vi "save log.vi"(4 "camera":bool, 5 "auto/man":bool, 6 "projector":bool, 7 "disc":bool, 8 "Error in":errorcluster, 10 "Case Num":u32, 11 "Disc Number":string="Disc 26") -> (0 "Error out":errorcluster)   [LabVIEW 2019, in "database.lvlib"]
uses:
  database.lvlib
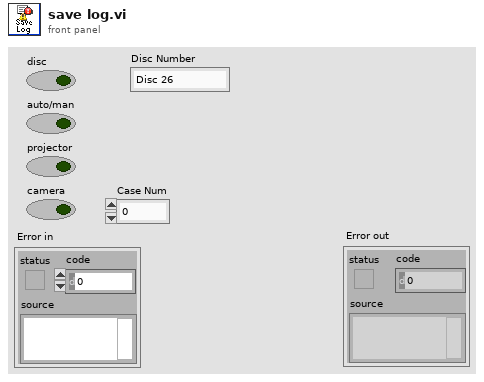
[diagram p1: front panel]
types:
  T1 = cluster{"f":string, "date/time string":string, "date/time string":string, "Disc Number":string}
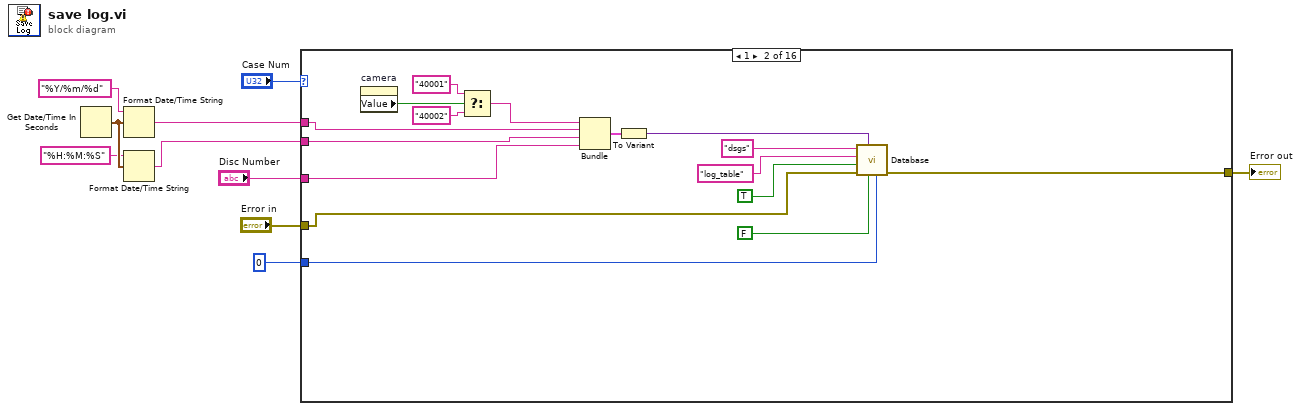
[diagram p0: block diagram]
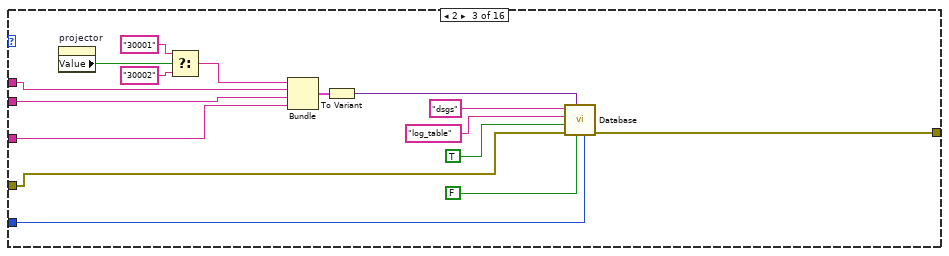
[diagram p3: hidden frame]
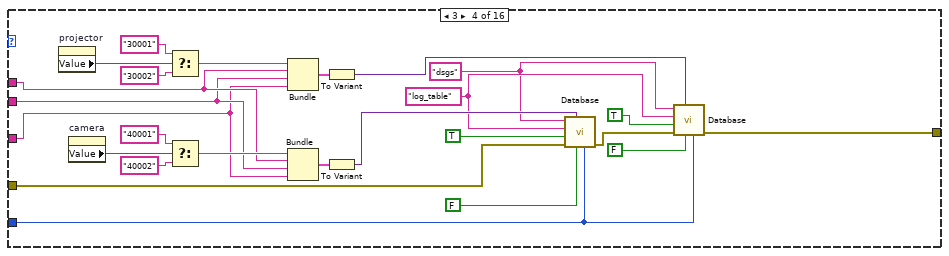
[diagram p4: hidden frame]
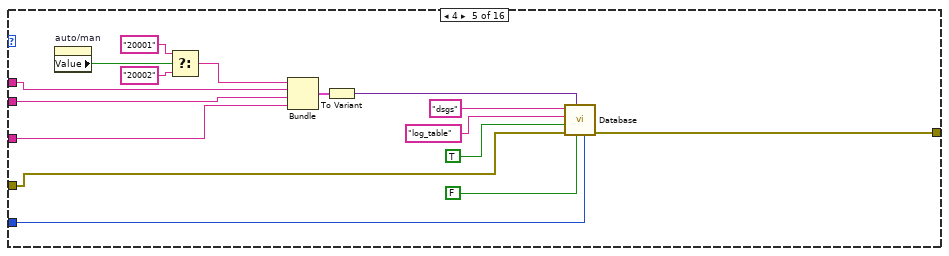
[diagram p5: hidden frame]
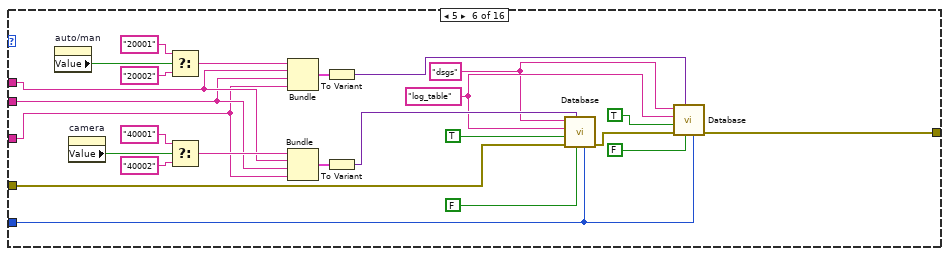
[diagram p6: hidden frame]
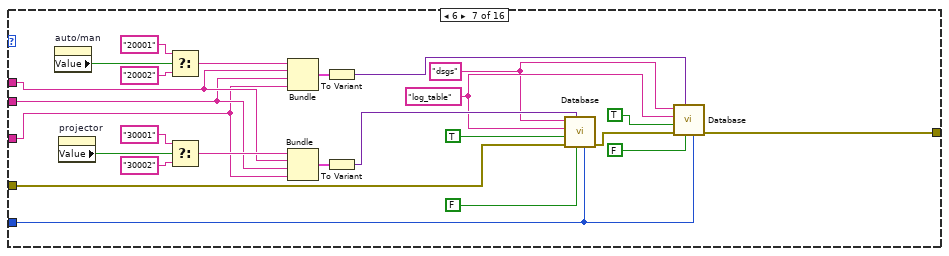
[diagram p7: hidden frame]
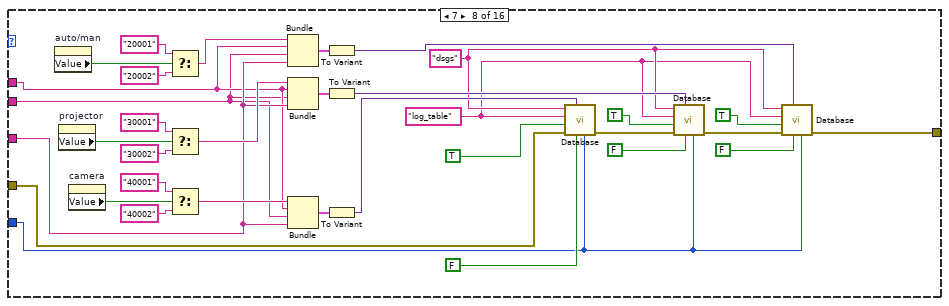
[diagram p8: hidden frame]
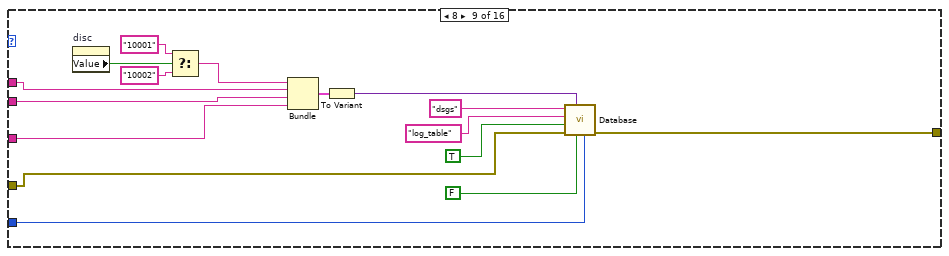
[diagram p9: hidden frame]
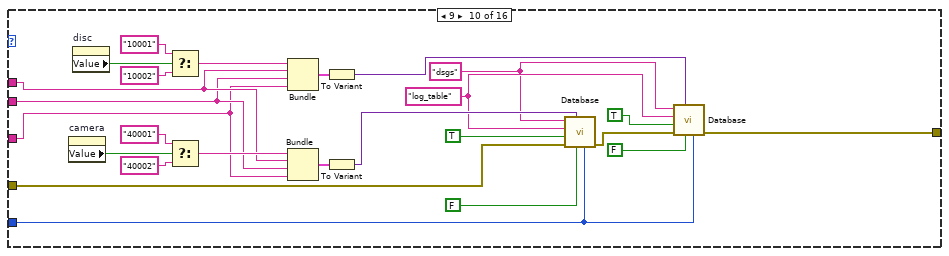
[diagram p10: hidden frame]
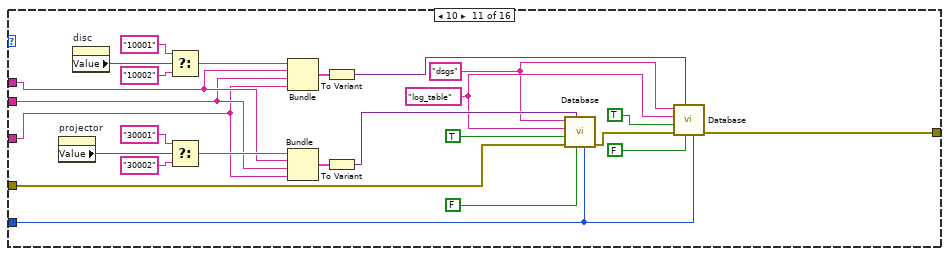
[diagram p11: hidden frame]
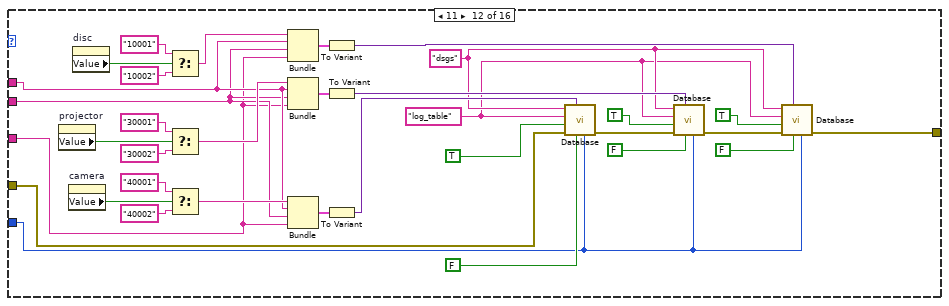
[diagram p12: hidden frame]
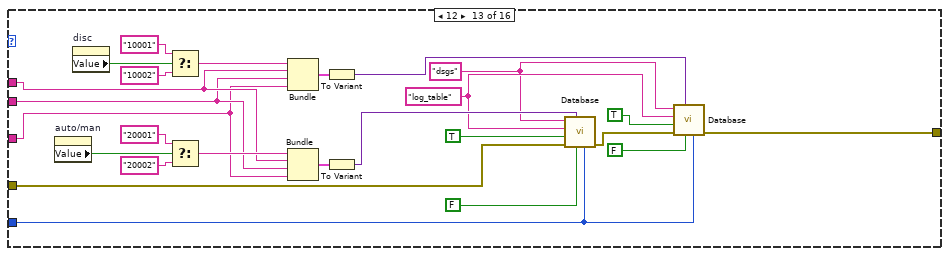
[diagram p13: hidden frame]
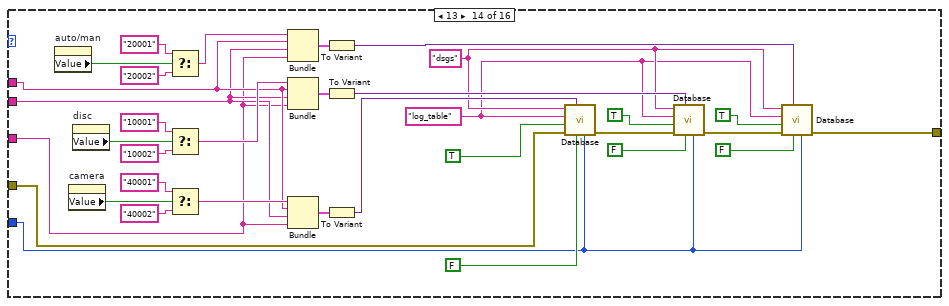
[diagram p14: hidden frame]
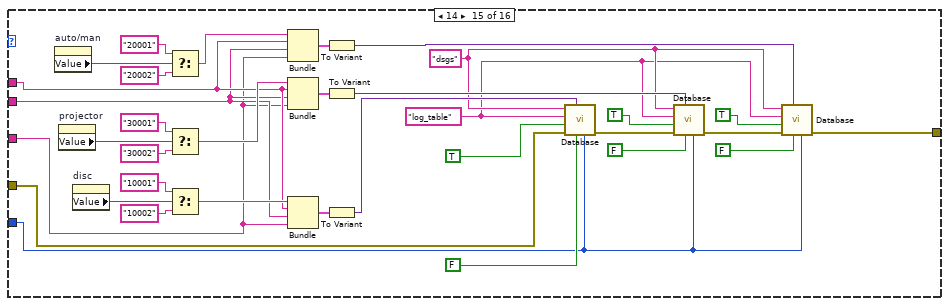
[diagram p15: hidden frame]
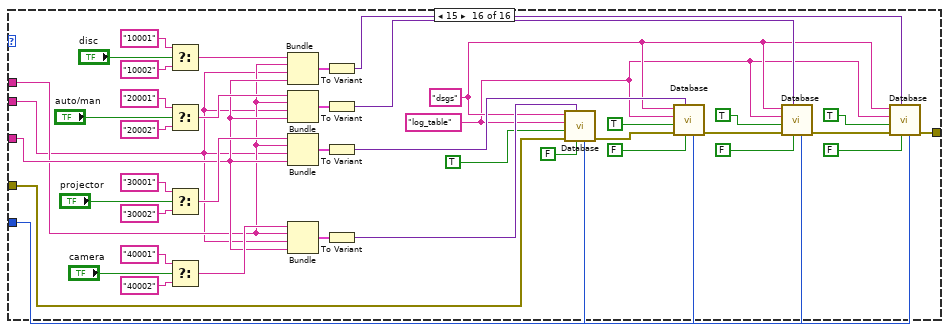
[diagram p16: hidden frame]
diagram:
  n1 = Get Date/Time In Seconds() -> (seconds since 1Jan1904=w6:timestamp)
  n2 = Format Date/Time String(time format string (%c)="%Y/%m/%d", seconds (now)=w6) -> (date/time string=w2:string)  [unwired: 1 in]
  n3 = Format Date/Time String(time format string (%c)="%H:%M:%S", seconds (now)=w6) -> (date/time string=w3:string)  [unwired: 1 in]
  n4 = case shown="1" "Case Num" {
    tunnel: "Error in" -> [w11 w24 w33 w61 w75 w92 w117 w153 w175 w192 w217 w243 w276 w302 w336 w381]
    tunnel: u64 0 ("Storage Time (Day) log") -> [_ w22 w32 w57 w74 w91 w116 w146 w174 w191 w216 w242 w275 w301 w335 w373]
    tunnel: [w11 w21 w34 w52 w73 w90 w115 w141 w173 w190 w215 w241 w274 w300 w334 w372] -> w7
    tunnel: w3 -> [_ w14 w29 w45 w70 w86 w111 w135 w170 w186 w211 w236 w270 w295 w329 w362]
    tunnel: w2 -> [_ w13 w30 w46 w71 w87 w112 w136 w171 w187 w212 w237 w271 w296 w330 w363]
    tunnel: "Disc Number" -> [_ w12 w28 w44 w69 w85 w110 w137 w169 w185 w210 w235 w269 w294 w328 w364]
    frame 0, Default {
    }
    frame 1 {
      n5 = property on="camera" class="Bool (strict)"() -> ("Value"=w15:bool)  [unwired: 2 in, 2 out]
      n6 = Select(t="40001" ("Table"), s=w15, f="40002") -> (s? t:f=w20:string)
      n7 = Bundle("f"=w20, "date/time string"=w13, "date/time string"=w14, "Disc Number"=w12) -> (w19:T1)  [unwired: 1 in]
      n8 = To Variant(anything=w19) -> (Variant=w18:variant)
      n9 = call "Database.vi"("Maximum Row"=w22, "Delete row?"=FALSE, "Data"=w18, "Error in"=w24, "Auto Increment ID?"=TRUE, "Table"="log_table", "Connection"="dsgs") -> ("Error out"=w21:errorcluster)  [unwired: 4 in]
    }
    frame 2 {
      n10 = property on="projector" class="Bool (strict)"() -> ("Value"=w31:bool)  [unwired: 2 in, 2 out]
      n11 = Select(t="30001" ("Table"), s=w31, f="30002") -> (s? t:f=w43:string)
      n12 = Bundle("f"=w43, "date/time string"=w30, "date/time string"=w29, "Disc Number"=w28) -> (w42:T1)  [unwired: 1 in]
      n13 = To Variant(anything=w42) -> (Variant=w41:variant)
      n14 = call "Database.vi"("Maximum Row"=w32, "Delete row?"=FALSE, "Data"=w41, "Error in"=w33, "Auto Increment ID?"=TRUE, "Table"="log_table", "Connection"="dsgs") -> ("Error out"=w34:errorcluster)  [unwired: 4 in]
    }
    frame 3 {
      w56 = "log_table" ("Table")
      w55 = "dsgs" ("Connection")
      n15 = property on="projector" class="Bool (strict)"() -> ("Value"=w48:bool)  [unwired: 2 in, 2 out]
      n16 = property on="camera" class="Bool (strict)"() -> ("Value"=w47:bool)  [unwired: 2 in, 2 out]
      n17 = Select(t="30001" ("Table"), s=w48, f="30002") -> (s? t:f=w51:string)
      n18 = Select(t="40001" ("Table"), s=w47, f="40002") -> (s? t:f=w68:string)
      n19 = Bundle("f"=w51, "date/time string"=w46, "date/time string"=w45, "Disc Number"=w44) -> (w50:T1)  [unwired: 1 in]
      n20 = Bundle("f"=w68, "date/time string"=w46, "date/time string"=w45, "Disc Number"=w44) -> (w67:T1)  [unwired: 1 in]
      n21 = To Variant(anything=w50) -> (Variant=w49:variant)
      n22 = To Variant(anything=w67) -> (Variant=w66:variant)
      n23 = call "Database.vi"("Maximum Row"=w57, "Delete row?"=FALSE, "Data"=w66, "Error in"=w61, "Auto Increment ID?"=TRUE, "Table"=w56, "Connection"=w55) -> ("Error out"=w60:errorcluster)  [unwired: 4 in]
      n24 = call "Database.vi"("Maximum Row"=w57, "Delete row?"=FALSE, "Data"=w49, "Error in"=w60, "Auto Increment ID?"=TRUE, "Table"=w56, "Connection"=w55) -> ("Error out"=w52:errorcluster)  [unwired: 4 in]
    }
    frame 4 {
      n25 = property on="auto/man" class="Bool (strict)"() -> ("Value"=w72:bool)  [unwired: 2 in, 2 out]
      n26 = Select(t="20001" ("Table"), s=w72, f="20002") -> (s? t:f=w84:string)
      n27 = Bundle("f"=w84, "date/time string"=w71, "date/time string"=w70, "Disc Number"=w69) -> (w83:T1)  [unwired: 1 in]
      n28 = To Variant(anything=w83) -> (Variant=w82:variant)
      n29 = call "Database.vi"("Maximum Row"=w74, "Delete row?"=FALSE, "Data"=w82, "Error in"=w75, "Auto Increment ID?"=TRUE, "Table"="log_table", "Connection"="dsgs") -> ("Error out"=w73:errorcluster)  [unwired: 4 in]
    }
    frame 5 {
      w99 = "log_table" ("Table")
      w98 = "dsgs" ("Connection")
      n30 = property on="auto/man" class="Bool (strict)"() -> ("Value"=w88:bool)  [unwired: 2 in, 2 out]
      n31 = property on="camera" class="Bool (strict)"() -> ("Value"=w89:bool)  [unwired: 2 in, 2 out]
      n32 = Select(t="20001" ("Table"), s=w88, f="20002") -> (s? t:f=w95:string)
      n33 = Select(t="40001" ("Table"), s=w89, f="40002") -> (s? t:f=w109:string)
      n34 = Bundle("f"=w95, "date/time string"=w87, "date/time string"=w86, "Disc Number"=w85) -> (w94:T1)  [unwired: 1 in]
      n35 = Bundle("f"=w109, "date/time string"=w87, "date/time string"=w86, "Disc Number"=w85) -> (w108:T1)  [unwired: 1 in]
      n36 = To Variant(anything=w94) -> (Variant=w93:variant)
      n37 = To Variant(anything=w108) -> (Variant=w107:variant)
      n38 = call "Database.vi"("Maximum Row"=w91, "Delete row?"=FALSE, "Data"=w107, "Error in"=w92, "Auto Increment ID?"=TRUE, "Table"=w99, "Connection"=w98) -> ("Error out"=w102:errorcluster)  [unwired: 4 in]
      n39 = call "Database.vi"("Maximum Row"=w91, "Delete row?"=FALSE, "Data"=w93, "Error in"=w102, "Auto Increment ID?"=TRUE, "Table"=w99, "Connection"=w98) -> ("Error out"=w90:errorcluster)  [unwired: 4 in]
    }
    frame 6 {
      w124 = "log_table" ("Table")
      w123 = "dsgs" ("Connection")
      n40 = property on="auto/man" class="Bool (strict)"() -> ("Value"=w113:bool)  [unwired: 2 in, 2 out]
      n41 = property on="projector" class="Bool (strict)"() -> ("Value"=w114:bool)  [unwired: 2 in, 2 out]
      n42 = Select(t="20001" ("Table"), s=w113, f="20002") -> (s? t:f=w120:string)
      n43 = Select(t="30001" ("Table"), s=w114, f="30002") -> (s? t:f=w134:string)
      n44 = Bundle("f"=w120, "date/time string"=w112, "date/time string"=w111, "Disc Number"=w110) -> (w119:T1)  [unwired: 1 in]
      n45 = Bundle("f"=w134, "date/time string"=w112, "date/time string"=w111, "Disc Number"=w110) -> (w133:T1)  [unwired: 1 in]
      n46 = To Variant(anything=w119) -> (Variant=w118:variant)
      n47 = To Variant(anything=w133) -> (Variant=w132:variant)
      n48 = call "Database.vi"("Maximum Row"=w116, "Delete row?"=FALSE, "Data"=w132, "Error in"=w117, "Auto Increment ID?"=TRUE, "Table"=w124, "Connection"=w123) -> ("Error out"=w127:errorcluster)  [unwired: 4 in]
      n49 = call "Database.vi"("Maximum Row"=w116, "Delete row?"=FALSE, "Data"=w118, "Error in"=w127, "Auto Increment ID?"=TRUE, "Table"=w124, "Connection"=w123) -> ("Error out"=w115:errorcluster)  [unwired: 4 in]
    }
    frame 7 {
      w143 = "log_table" ("Table")
      w144 = "dsgs" ("Connection")
      n50 = property on="auto/man" class="Bool (strict)"() -> ("Value"=w140:bool)  [unwired: 2 in, 2 out]
      n51 = property on="projector" class="Bool (strict)"() -> ("Value"=w139:bool)  [unwired: 2 in, 2 out]
      n52 = property on="camera" class="Bool (strict)"() -> ("Value"=w138:bool)  [unwired: 2 in, 2 out]
      n53 = Select(t="20001" ("Table"), s=w140, f="20002") -> (s? t:f=w150:string)
      n54 = Select(t="30001" ("Table"), s=w139, f="30002") -> (s? t:f=w156:string)
      n55 = Select(t="40001" ("Table"), s=w138, f="40002") -> (s? t:f=w168:string)
      n56 = Bundle("f"=w150, "date/time string"=w136, "date/time string"=w135, "Disc Number"=w137) -> (w151:T1)  [unwired: 1 in]
      n57 = Bundle("f"=w156, "date/time string"=w136, "date/time string"=w135, "Disc Number"=w137) -> (w155:T1)  [unwired: 1 in]
      n58 = Bundle("f"=w168, "date/time string"=w136, "date/time string"=w135, "Disc Number"=w137) -> (w167:T1)  [unwired: 1 in]
      n59 = To Variant(anything=w151) -> (Variant=w152:variant)
      n60 = To Variant(anything=w155) -> (Variant=w154:variant)
      n61 = To Variant(anything=w167) -> (Variant=w166:variant)
      n62 = call "Database.vi"("Maximum Row"=w146, "Delete row?"=FALSE, "Data"=w166, "Error in"=w153, "Auto Increment ID?"=TRUE, "Table"=w143, "Connection"=w144) -> ("Error out"=w161:errorcluster)  [unwired: 4 in]
      n63 = call "Database.vi"("Maximum Row"=w146, "Delete row?"=FALSE, "Data"=w154, "Error in"=w161, "Auto Increment ID?"=TRUE, "Table"=w143, "Connection"=w144) -> ("Error out"=w145:errorcluster)  [unwired: 4 in]
      n64 = call "Database.vi"("Maximum Row"=w146, "Delete row?"=FALSE, "Data"=w152, "Error in"=w145, "Auto Increment ID?"=TRUE, "Table"=w143, "Connection"=w144) -> ("Error out"=w141:errorcluster)  [unwired: 4 in]
    }
    frame 8 {
      n65 = property on="disc" class="Bool (strict)"() -> ("Value"=w172:bool)  [unwired: 2 in, 2 out]
      n66 = Select(t="10001" ("Table"), s=w172, f="10002") -> (s? t:f=w184:string)
      n67 = Bundle("f"=w184, "date/time string"=w171, "date/time string"=w170, "Disc Number"=w169) -> (w183:T1)  [unwired: 1 in]
      n68 = To Variant(anything=w183) -> (Variant=w182:variant)
      n69 = call "Database.vi"("Maximum Row"=w174, "Delete row?"=FALSE, "Data"=w182, "Error in"=w175, "Auto Increment ID?"=TRUE, "Table"="log_table", "Connection"="dsgs") -> ("Error out"=w173:errorcluster)  [unwired: 4 in]
    }
    frame 9 {
      w199 = "log_table" ("Table")
      w198 = "dsgs" ("Connection")
      n70 = property on="camera" class="Bool (strict)"() -> ("Value"=w188:bool)  [unwired: 2 in, 2 out]
      n71 = property on="disc" class="Bool (strict)"() -> ("Value"=w189:bool)  [unwired: 2 in, 2 out]
      n72 = Select(t="10001" ("Table"), s=w189, f="10002") -> (s? t:f=w195:string)
      n73 = Select(t="40001" ("Table"), s=w188, f="40002") -> (s? t:f=w209:string)
      n74 = Bundle("f"=w195, "date/time string"=w187, "date/time string"=w186, "Disc Number"=w185) -> (w194:T1)  [unwired: 1 in]
      n75 = Bundle("f"=w209, "date/time string"=w187, "date/time string"=w186, "Disc Number"=w185) -> (w208:T1)  [unwired: 1 in]
      n76 = To Variant(anything=w194) -> (Variant=w193:variant)
      n77 = To Variant(anything=w208) -> (Variant=w207:variant)
      n78 = call "Database.vi"("Maximum Row"=w191, "Delete row?"=FALSE, "Data"=w207, "Error in"=w192, "Auto Increment ID?"=TRUE, "Table"=w199, "Connection"=w198) -> ("Error out"=w202:errorcluster)  [unwired: 4 in]
      n79 = call "Database.vi"("Maximum Row"=w191, "Delete row?"=FALSE, "Data"=w193, "Error in"=w202, "Auto Increment ID?"=TRUE, "Table"=w199, "Connection"=w198) -> ("Error out"=w190:errorcluster)  [unwired: 4 in]
    }
    frame 10 {
      w224 = "log_table" ("Table")
      w223 = "dsgs" ("Connection")
      n80 = property on="projector" class="Bool (strict)"() -> ("Value"=w213:bool)  [unwired: 2 in, 2 out]
      n81 = property on="disc" class="Bool (strict)"() -> ("Value"=w214:bool)  [unwired: 2 in, 2 out]
      n82 = Select(t="10001" ("Table"), s=w214, f="10002") -> (s? t:f=w220:string)
      n83 = Select(t="30001" ("Table"), s=w213, f="30002") -> (s? t:f=w234:string)
      n84 = Bundle("f"=w220, "date/time string"=w212, "date/time string"=w211, "Disc Number"=w210) -> (w219:T1)  [unwired: 1 in]
      n85 = Bundle("f"=w234, "date/time string"=w212, "date/time string"=w211, "Disc Number"=w210) -> (w233:T1)  [unwired: 1 in]
      n86 = To Variant(anything=w219) -> (Variant=w218:variant)
      n87 = To Variant(anything=w233) -> (Variant=w232:variant)
      n88 = call "Database.vi"("Maximum Row"=w216, "Delete row?"=FALSE, "Data"=w232, "Error in"=w217, "Auto Increment ID?"=TRUE, "Table"=w224, "Connection"=w223) -> ("Error out"=w227:errorcluster)  [unwired: 4 in]
      n89 = call "Database.vi"("Maximum Row"=w216, "Delete row?"=FALSE, "Data"=w218, "Error in"=w227, "Auto Increment ID?"=TRUE, "Table"=w224, "Connection"=w223) -> ("Error out"=w215:errorcluster)  [unwired: 4 in]
    }
    frame 11 {
      w245 = "log_table" ("Table")
      w246 = "dsgs" ("Connection")
      n90 = property on="projector" class="Bool (strict)"() -> ("Value"=w239:bool)  [unwired: 2 in, 2 out]
      n91 = property on="camera" class="Bool (strict)"() -> ("Value"=w238:bool)  [unwired: 2 in, 2 out]
      n92 = property on="disc" class="Bool (strict)"() -> ("Value"=w240:bool)  [unwired: 2 in, 2 out]
      n93 = Select(t="10001" ("Table"), s=w240, f="10002") -> (s? t:f=w251:string)
      n94 = Select(t="30001" ("Table"), s=w239, f="30002") -> (s? t:f=w256:string)
      n95 = Select(t="40001" ("Table"), s=w238, f="40002") -> (s? t:f=w268:string)
      n96 = Bundle("f"=w251, "date/time string"=w237, "date/time string"=w236, "Disc Number"=w235) -> (w252:T1)  [unwired: 1 in]
      n97 = Bundle("f"=w256, "date/time string"=w237, "date/time string"=w236, "Disc Number"=w235) -> (w255:T1)  [unwired: 1 in]
      n98 = Bundle("f"=w268, "date/time string"=w237, "date/time string"=w236, "Disc Number"=w235) -> (w267:T1)  [unwired: 1 in]
      n99 = To Variant(anything=w252) -> (Variant=w253:variant)
      n100 = To Variant(anything=w255) -> (Variant=w254:variant)
      n101 = To Variant(anything=w267) -> (Variant=w266:variant)
      n102 = call "Database.vi"("Maximum Row"=w242, "Delete row?"=FALSE, "Data"=w266, "Error in"=w243, "Auto Increment ID?"=TRUE, "Table"=w245, "Connection"=w246) -> ("Error out"=w261:errorcluster)  [unwired: 4 in]
      n103 = call "Database.vi"("Maximum Row"=w242, "Delete row?"=FALSE, "Data"=w254, "Error in"=w261, "Auto Increment ID?"=TRUE, "Table"=w245, "Connection"=w246) -> ("Error out"=w247:errorcluster)  [unwired: 4 in]
      n104 = call "Database.vi"("Maximum Row"=w242, "Delete row?"=FALSE, "Data"=w253, "Error in"=w247, "Auto Increment ID?"=TRUE, "Table"=w245, "Connection"=w246) -> ("Error out"=w241:errorcluster)  [unwired: 4 in]
    }
    frame 12 {
      w283 = "log_table" ("Table")
      w282 = "dsgs" ("Connection")
      n105 = property on="auto/man" class="Bool (strict)"() -> ("Value"=w273:bool)  [unwired: 2 in, 2 out]
      n106 = property on="disc" class="Bool (strict)"() -> ("Value"=w272:bool)  [unwired: 2 in, 2 out]
      n107 = Select(t="10001" ("Table"), s=w272, f="10002") -> (s? t:f=w279:string)
      n108 = Select(t="20001" ("Table"), s=w273, f="20002") -> (s? t:f=w293:string)
      n109 = Bundle("f"=w279, "date/time string"=w271, "date/time string"=w270, "Disc Number"=w269) -> (w278:T1)  [unwired: 1 in]
      n110 = Bundle("f"=w293, "date/time string"=w271, "date/time string"=w270, "Disc Number"=w269) -> (w292:T1)  [unwired: 1 in]
      n111 = To Variant(anything=w278) -> (Variant=w277:variant)
      n112 = To Variant(anything=w292) -> (Variant=w291:variant)
      n113 = call "Database.vi"("Maximum Row"=w275, "Delete row?"=FALSE, "Data"=w291, "Error in"=w276, "Auto Increment ID?"=TRUE, "Table"=w283, "Connection"=w282) -> ("Error out"=w286:errorcluster)  [unwired: 4 in]
      n114 = call "Database.vi"("Maximum Row"=w275, "Delete row?"=FALSE, "Data"=w277, "Error in"=w286, "Auto Increment ID?"=TRUE, "Table"=w283, "Connection"=w282) -> ("Error out"=w274:errorcluster)  [unwired: 4 in]
    }
    frame 13 {
      w304 = "log_table" ("Table")
      w305 = "dsgs" ("Connection")
      n115 = property on="auto/man" class="Bool (strict)"() -> ("Value"=w298:bool)  [unwired: 2 in, 2 out]
      n116 = property on="camera" class="Bool (strict)"() -> ("Value"=w299:bool)  [unwired: 2 in, 2 out]
      n117 = property on="disc" class="Bool (strict)"() -> ("Value"=w297:bool)  [unwired: 2 in, 2 out]
      n118 = Select(t="20001" ("Table"), s=w298, f="20002") -> (s? t:f=w310:string)
      n119 = Select(t="10001" ("Table"), s=w297, f="10002") -> (s? t:f=w315:string)
      n120 = Select(t="40001" ("Table"), s=w299, f="40002") -> (s? t:f=w327:string)
      n121 = Bundle("f"=w310, "date/time string"=w296, "date/time string"=w295, "Disc Number"=w294) -> (w311:T1)  [unwired: 1 in]
      n122 = Bundle("f"=w315, "date/time string"=w296, "date/time string"=w295, "Disc Number"=w294) -> (w314:T1)  [unwired: 1 in]
      n123 = Bundle("f"=w327, "date/time string"=w296, "date/time string"=w295, "Disc Number"=w294) -> (w326:T1)  [unwired: 1 in]
      n124 = To Variant(anything=w311) -> (Variant=w312:variant)
      n125 = To Variant(anything=w314) -> (Variant=w313:variant)
      n126 = To Variant(anything=w326) -> (Variant=w325:variant)
      n127 = call "Database.vi"("Maximum Row"=w301, "Delete row?"=FALSE, "Data"=w325, "Error in"=w302, "Auto Increment ID?"=TRUE, "Table"=w304, "Connection"=w305) -> ("Error out"=w320:errorcluster)  [unwired: 4 in]
      n128 = call "Database.vi"("Maximum Row"=w301, "Delete row?"=FALSE, "Data"=w313, "Error in"=w320, "Auto Increment ID?"=TRUE, "Table"=w304, "Connection"=w305) -> ("Error out"=w306:errorcluster)  [unwired: 4 in]
      n129 = call "Database.vi"("Maximum Row"=w301, "Delete row?"=FALSE, "Data"=w312, "Error in"=w306, "Auto Increment ID?"=TRUE, "Table"=w304, "Connection"=w305) -> ("Error out"=w300:errorcluster)  [unwired: 4 in]
    }
    frame 14 {
      w338 = "log_table" ("Table")
      w339 = "dsgs" ("Connection")
      n130 = property on="auto/man" class="Bool (strict)"() -> ("Value"=w332:bool)  [unwired: 2 in, 2 out]
      n131 = property on="projector" class="Bool (strict)"() -> ("Value"=w333:bool)  [unwired: 2 in, 2 out]
      n132 = property on="disc" class="Bool (strict)"() -> ("Value"=w331:bool)  [unwired: 2 in, 2 out]
      n133 = Select(t="20001" ("Table"), s=w332, f="20002") -> (s? t:f=w344:string)
      n134 = Select(t="30001" ("Table"), s=w333, f="30002") -> (s? t:f=w349:string)
      n135 = Select(t="10001" ("Table"), s=w331, f="10002") -> (s? t:f=w361:string)
      n136 = Bundle("f"=w344, "date/time string"=w330, "date/time string"=w329, "Disc Number"=w328) -> (w345:T1)  [unwired: 1 in]
      n137 = Bundle("f"=w349, "date/time string"=w330, "date/time string"=w329, "Disc Number"=w328) -> (w348:T1)  [unwired: 1 in]
      n138 = Bundle("f"=w361, "date/time string"=w330, "date/time string"=w329, "Disc Number"=w328) -> (w360:T1)  [unwired: 1 in]
      n139 = To Variant(anything=w345) -> (Variant=w346:variant)
      n140 = To Variant(anything=w348) -> (Variant=w347:variant)
      n141 = To Variant(anything=w360) -> (Variant=w359:variant)
      n142 = call "Database.vi"("Maximum Row"=w335, "Delete row?"=FALSE, "Data"=w359, "Error in"=w336, "Auto Increment ID?"=TRUE, "Table"=w338, "Connection"=w339) -> ("Error out"=w354:errorcluster)  [unwired: 4 in]
      n143 = call "Database.vi"("Maximum Row"=w335, "Delete row?"=FALSE, "Data"=w347, "Error in"=w354, "Auto Increment ID?"=TRUE, "Table"=w338, "Connection"=w339) -> ("Error out"=w340:errorcluster)  [unwired: 4 in]
      n144 = call "Database.vi"("Maximum Row"=w335, "Delete row?"=FALSE, "Data"=w346, "Error in"=w340, "Auto Increment ID?"=TRUE, "Table"=w338, "Connection"=w339) -> ("Error out"=w334:errorcluster)  [unwired: 4 in]
    }
    frame 15 {
      w369 = "log_table" ("Table")
      w370 = "dsgs" ("Connection")
      n145 = Select(t="10001" ("Table"), s="disc", f="10002") -> (s? t:f=w376:string)
      n146 = Select(t="20001" ("Table"), s="auto/man", f="20002") -> (s? t:f=w387:string)
      n147 = Select(t="30001" ("Table"), s="projector", f="30002") -> (s? t:f=w392:string)
      n148 = Select(t="40001" ("Table"), s="camera", f="40002") -> (s? t:f=w404:string)
      n149 = Bundle("f"=w376, "date/time string"=w363, "date/time string"=w362, "Disc Number"=w364) -> (w375:T1)  [unwired: 1 in]
      n150 = Bundle("f"=w387, "date/time string"=w363, "date/time string"=w362, "Disc Number"=w364) -> (w388:T1)  [unwired: 1 in]
      n151 = Bundle("f"=w392, "date/time string"=w363, "date/time string"=w362, "Disc Number"=w364) -> (w391:T1)  [unwired: 1 in]
      n152 = Bundle("f"=w404, "date/time string"=w363, "date/time string"=w362, "Disc Number"=w364) -> (w403:T1)  [unwired: 1 in]
      n153 = To Variant(anything=w375) -> (Variant=w374:variant)
      n154 = To Variant(anything=w388) -> (Variant=w389:variant)
      n155 = To Variant(anything=w391) -> (Variant=w390:variant)
      n156 = To Variant(anything=w403) -> (Variant=w402:variant)
      n157 = call "Database.vi"("Maximum Row"=w373, "Delete row?"=FALSE, "Data"=w402, "Error in"=w381, "Auto Increment ID?"=TRUE, "Table"=w369, "Connection"=w370) -> ("Error out"=w397:errorcluster)  [unwired: 4 in]
      n158 = call "Database.vi"("Maximum Row"=w373, "Delete row?"=FALSE, "Data"=w390, "Error in"=w397, "Auto Increment ID?"=TRUE, "Table"=w369, "Connection"=w370) -> ("Error out"=w383:errorcluster)  [unwired: 4 in]
      n159 = call "Database.vi"("Maximum Row"=w373, "Delete row?"=FALSE, "Data"=w389, "Error in"=w383, "Auto Increment ID?"=TRUE, "Table"=w369, "Connection"=w370) -> ("Error out"=w371:errorcluster)  [unwired: 4 in]
      n160 = call "Database.vi"("Maximum Row"=w373, "Delete row?"=FALSE, "Data"=w374, "Error in"=w371, "Auto Increment ID?"=TRUE, "Table"=w369, "Connection"=w370) -> ("Error out"=w372:errorcluster)  [unwired: 4 in]
    }
  }
  "Error out" <- w7
